vi "SpanConfig.vi"(8 "error in (no error)":errorcluster, 9 "Span (Hz)":dbl, 10 "Center Frequency (Hz)":dbl, 11 "SpecA_MXA in":refnum<class "SpecA_MXA.lvclass">) -> (0 "error out":errorcluster, 3 "SpecA_MXA out":refnum<class "SpecA_MXA.lvclass">)   [LabVIEW 2014, in "SpecA_MXA.lvclass"]
uses:
  SpecA_MXA.lvclass
  Instrument.lvclass
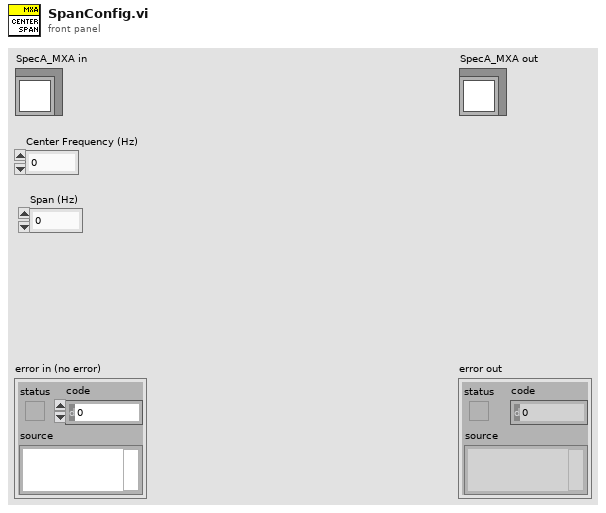
[diagram p1: front panel]
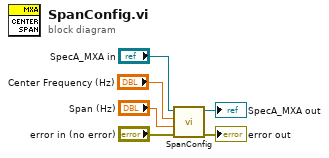
[diagram p0: block diagram]
diagram:
  n1 = call-parent "SpanConfig.vi"("error in (no error)"="error in (no error)", "Span (Hz)"="Span (Hz)", "Center Frequency (Hz)"="Center Frequency (Hz)", "Instrument in"="SpecA_MXA in") -> ("error out"=→"error out":errorcluster, "Instrument out"=→"SpecA_MXA out":refnum<class "SpecA_MXA.lvclass">)  [unwired: 6 in]
